vi "test-quintic-spline-00.vi"() -> (3 "Test Passed":bool)   [LabVIEW 2019]
uses:
  <vilib>/Rock Robotics/WPI/ThirdParty/JAS_Junk/TrajLib/POSEwCURVATURE.ctl
  <vilib>/Rock Robotics/WPI/ThirdParty/JAS_Junk/TrajLib/POSE2D.ctl
  <vilib>/Rock Robotics/WPI/ThirdParty/JAS_Junk/TrajLib/TRANSLATION2D.ctl
  <vilib>/Rock Robotics/WPI/ThirdParty/JAS_Junk/TrajLib/ROTATION2D.ctl
  <vilib>/Rock Robotics/WPI/ThirdParty/JAS_Junk/TrajLib/Rotation2d_CreateAngle.vi
  <vilib>/Rock Robotics/WPI/ThirdParty/JAS_Junk/TrajLib/Translation2d_Create.vi
  <vilib>/Rock Robotics/WPI/ThirdParty/JAS_Junk/TrajLib/Util_CalcDist.vi
  <vilib>/Rock Robotics/WPI/ThirdParty/JAS_Junk/TrajLib/Trajectory_Library.lvlib
panel:
  out "XY Graph":cluster{dbl[], dbl[]}(graph)
  out "Numb\nWaypoints":i32
  out "All Interior \nwayPoints\nFound (True)":bool
  out "end rot = 0":dbl
  out "end y = 0":dbl
  out "end x = 0":dbl
  out "start rot = 0":dbl
  out "start y = 0":dbl
  out "start x = 0":dbl
  out "max dtheta < 0.0872":dbl
  out "max dy < 0.00127":dbl
  out "max dx  < 0.127":dbl
  out "Overall Error":errorcluster
  out "Elements":i32
  out "Create Spline Error":errorcluster
  out "SplinePoses\nWCurve":T1[](array[typedef]) {"POSE"."ROTATION"."SIN" format="%13.4f"; "POSE"."ROTATION"."COS" format="%13.4f"; "POSE"."ROTATION"."VALUE" format="%13.4f"; "POSE"."TRANSLATION"."Y" format="%14.3f"; "POSE"."TRANSLATION"."X" format="%14.3f"}
  out "Elapsed Time":dbl
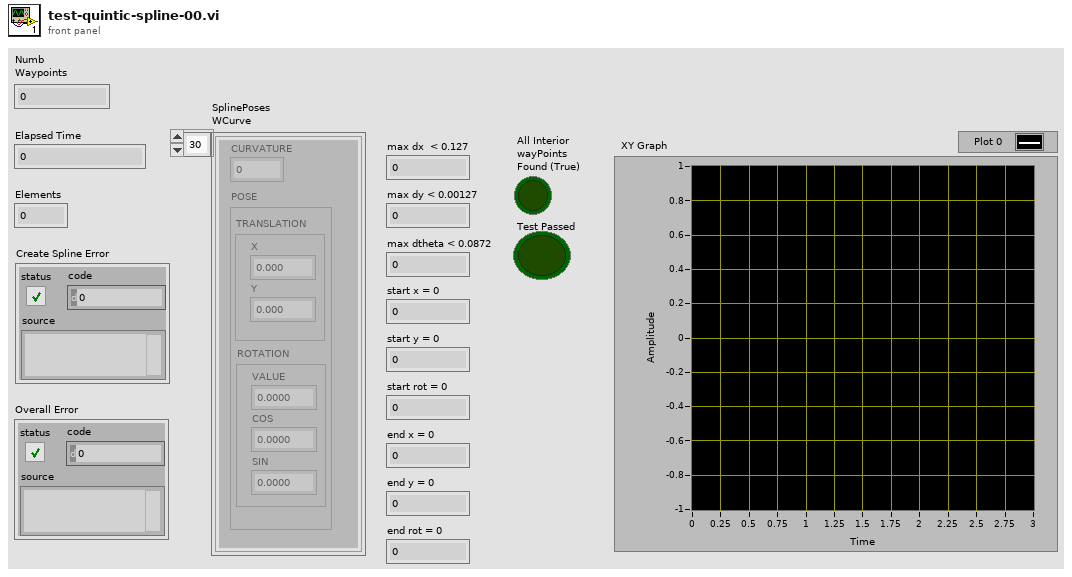
[diagram p1: front panel]
types:
  T1 = typedef "Trajectory_Library.lvlib/POSEwCURVATURE.ctl" = cluster{"CURVATURE":dbl, "POSE":T2}
  T2 = typedef "Trajectory_Library.lvlib/POSE2D.ctl" = cluster{"TRANSLATION":T3, "ROTATION":T4}
  T3 = typedef "Trajectory_Library.lvlib/TRANSLATION2D.ctl" = cluster{"X":dbl, "Y":dbl}
  T4 = typedef "Trajectory_Library.lvlib/ROTATION2D.ctl" = cluster{"VALUE":dbl, "COS":dbl, "SIN":dbl}
  T5 = typedef "Trajectory_Library.lvlib/SPLINE.ctl" = cluster{"Degree":i32, "Coefficients":T6}
  T6 = typedef "NI_Matrix.lvlib/RealMatrix.ctl" = dbl[][]
  T7 = typedef "Trajectory_Library.lvlib/TWIST2D.ctl" = cluster{"dX":dbl, "dY":dbl, "dTHETA":dbl}
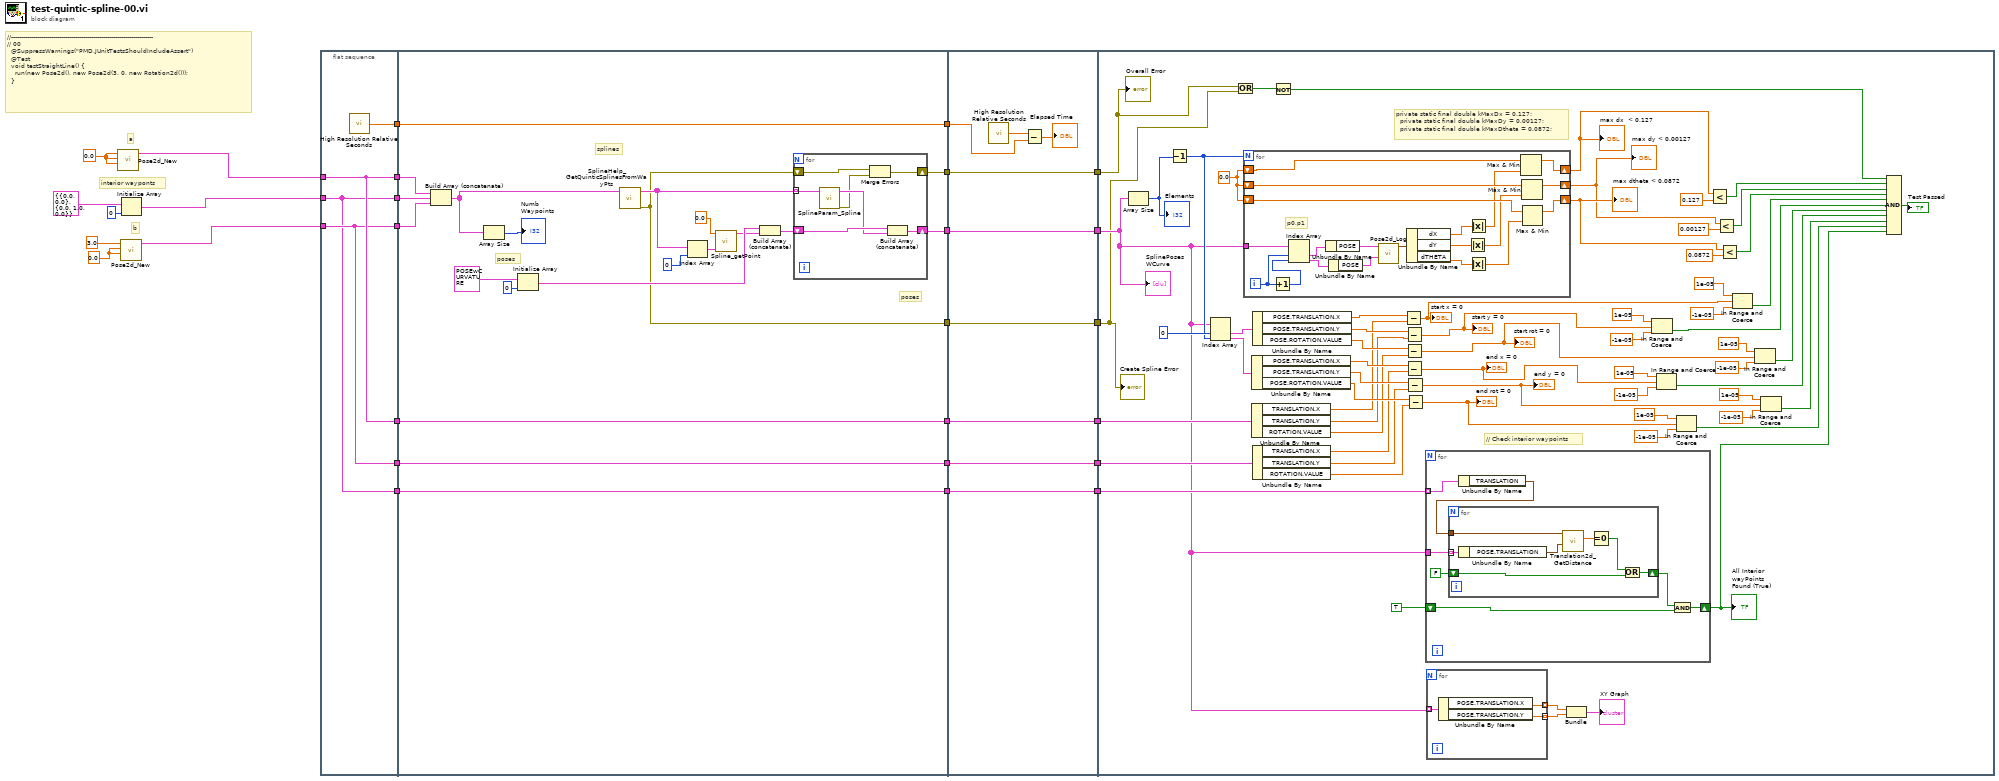
[diagram p0: block diagram]
diagram:
  w26 = 0.0 ("Y")
  w28 = 0.0 ("X")
  # "interior wayponts"
  # "b"
  # "a"
  # "//-----------------------------------------------------------------------\n// 00\n  @SuppressWarnings(\"PMD.JUnitTestsShouldIncludeAssert\")\n  @Test\n  void testStraightLine() {\n    run(new Pose2d(), new Pose2d(3, 0, new Rotation2d()));\n  }"
  n1 = call <vilib>:"Pose2d_New.vi"("Heading"=w28, "Y"=w28, "X"=w28) -> ("out POSe"=w25:T2)  [unwired: 8 in]
  n2 = call <vilib>:"Pose2d_New.vi"("Heading"=w26, "Y"=w26, "X"=3.0) -> ("out POSe"=w23:T2)  [unwired: 8 in]
  n3 = Initialize Array(T2 {"TRANSLATION"={"X"=0.0, "Y"=0.0}, "ROTATION"={"VALUE"=0.0, "COS"=1.0, "SIN"=0.0}} ("POSE"), 0 ("dimension size")) -> (w2:T2[])
  n4 = flat-sequence {
    tunnel: w25 -> [w31]
    tunnel: [w31] -> w24
    tunnel: w23 -> [w30]
    tunnel: [w30] -> w22
    tunnel: [w32] -> w21
    tunnel: [w31] -> w13
    tunnel: [w30] -> w10
    tunnel: [w29] -> w5
    tunnel: w2 -> [w29]
    tunnel: [w29] -> w1
    tunnel: w24 -> [w37]
    tunnel: w22 -> [w36]
    tunnel: [w53] -> w20
    tunnel: w21 -> [w53]
    tunnel: [w43] -> w19
    tunnel: [w42] -> w17
    tunnel: [w41] -> w15
    tunnel: w13 -> [w40]
    tunnel: [w40] -> w12
    tunnel: w10 -> [w39]
    tunnel: [w39] -> w9
    tunnel: [w38] -> w6
    tunnel: w5 -> [w38]
    tunnel: w1 -> [w35]
    tunnel: w20 -> [w69]
    tunnel: w19 -> [w68]
    tunnel: [w68] -> w18
    tunnel: w17 -> [w67]
    tunnel: [w67] -> w16
    tunnel: w15 -> [w66]
    tunnel: [w66] -> w14
    tunnel: w12 -> [w63]
    tunnel: [w63] -> w11
    tunnel: w9 -> [w62]
    tunnel: [w62] -> w8
    tunnel: [w61] -> w7
    tunnel: w6 -> [w61]
    tunnel: w18 -> [w110]
    tunnel: w16 -> [w97]
    tunnel: w14 -> [w96]
    tunnel: w11 -> [w132]
    tunnel: w8 -> [w131]
    tunnel: w7 -> [w114]
    frame #0 {
      n5 = call <vilib>:"High Resolution Relative Seconds.vi"() -> ("relative seconds"=w32:dbl)
    }
    frame #1 {
      # "poses"
      # "poses"
      # "splines"
      n6 = Build Array (concatenate)(w37, w35, w36) -> (w33:T2[])
      n7 = Array Size(array=w33) -> (size(s)=→"Numb\nWaypoints":i32)
      n8 = Initialize Array(T1 {"CURVATURE"=0.0, "POSE"={"TRANSLATION"={"X"=0.0, "Y"=0.0}, "ROTATION"={"VALUE"=0.0, "COS"=1.0, "SIN"=0.0}}} ("POSEwCURVATURE"), 0 ("dimension size")) -> (w47:T1[])
      n9 = call <vilib>:"SplineHelp_GetQuinticSplinesFromWayPts.vi"("WayPoints"=w33) -> ("out Error"=w42:errorcluster, "Splines"=w44:T5[])  [unwired: 9 in]
      n10 = Index Array(array=w44, index=0) -> (element=w49:T5)
      n11 = call <vilib>:"Spline_getPoint.vi"("inputSPLINE"=w49, "Time"=0.0) -> ("POSEwCURVATURE"=w46:T1)  [unwired: 9 in]
      n12 = Build Array (concatenate)(w47, w46) -> (w45:T1[])
      n13 = for {
        shift-right: [w57] -> w43
        shift-left: w45 -> [w59]
        tunnel: w44 -> [w60] mode=indexing
        shift-right: [w55] -> w41
        shift-left: w42 -> [w56]
        n14 = call <vilib>:"SplineParam_Spline.vi"("inputSPLINE"=w60) -> ("error out"=w54:errorcluster, "outputPOSEwCURVATURE"=w58:T1[])  [unwired: 9 in]
        n15 = Merge Errors(w56, w54) -> (w55:errorcluster)
        n16 = Build Array (concatenate)(w59, w58) -> (w57:T1[])
      }
    }
    frame #2 {
      n17 = call <vilib>:"High Resolution Relative Seconds.vi"() -> ("relative seconds"=w64:dbl)
      n18 = Subtract(x=w64, y=w69) -> (x-y=→"Elapsed Time":dbl)
    }
    frame #3 {
      w133 = 0.0
      # "// Check interior waypoints"
      # "private static final double kMaxDx = 0.127;\n  private static final double kMaxDy = 0.00127;\n  private static final double kMaxDtheta = 0.0872;"
      n19 = Array Size(array=w110) -> (size(s)=w134:i32)
      "Elements" <- w134
      n20 = Decrement(x=w134) -> (x-1=w129:i32)
      n21 = Index Array(array=w110, index #1=0 ("index"), index #2=w129) -> (element #1=w128:T1, element #2=w127:T1)
      n22 = Or(x=w96, y=w97) -> (x .or. y?=w98:bool)
      n23 = for {
        N: w129 -> [_]
        tunnel: w110 -> [w169]
        shift-right: [w160] -> w102
        shift-left: w133 -> [w157]
        shift-right: [w158] -> w104
        shift-left: w133 -> [w155]
        shift-right: [w159] -> w103
        shift-left: w133 -> [w156]
        i -> [w171]
        # "p0,p1"
        n24 = Increment(x=w171) -> (x+1=w170:i32)
        n25 = Index Array(array=w169, index #1=w171, index #2=w170) -> (element #1=w168:T1, element #2=w167:T1)
        n26 = Unbundle By Name(w168) -> ("POSE"=w166:T2)
        n27 = Unbundle By Name(w167) -> ("POSE"=w165:T2)
        n28 = call <vilib>:"Pose2d_Log.vi"("end POSE"=w165, "in POSE"=w166) -> ("out TWIST"=w164:T7)  [unwired: 9 in]
        n29 = Unbundle By Name(w164) -> ("dX"=w161:dbl, "dY"=w162:dbl, "dTHETA"=w163:dbl)
        n30 = Absolute Value(x=w162) -> (abs(x)=w153:dbl)
        n31 = Absolute Value(x=w161) -> (abs(x)=w154:dbl)
        n32 = Absolute Value(x=w163) -> (abs(x)=w152:dbl)
        n33 = Max & Min(x=w157, y=w154) -> (max(x,y)=w160:dbl)  [unwired: 1 out]
        n34 = Max & Min(x=w156, y=w153) -> (max(x,y)=w159:dbl)  [unwired: 1 out]
        n35 = Max & Min(x=w155, y=w152) -> (max(x,y)=w158:dbl)  [unwired: 1 out]
      }
      "max dx  < 0.127" <- w102
      "max dy < 0.00127" <- w103
      "max dtheta < 0.0872" <- w104
      n36 = Unbundle By Name(w127) -> ("POSE.TRANSLATION.X"=w123:dbl, "POSE.TRANSLATION.Y"=w122:dbl, "POSE.ROTATION.VALUE"=w121:dbl)
      n37 = Unbundle By Name(w132) -> ("TRANSLATION.X"=w120:dbl, "TRANSLATION.Y"=w119:dbl, "ROTATION.VALUE"=w118:dbl)
      n38 = Unbundle By Name(w128) -> ("POSE.TRANSLATION.X"=w126:dbl, "POSE.TRANSLATION.Y"=w125:dbl, "POSE.ROTATION.VALUE"=w124:dbl)
      n39 = Unbundle By Name(w131) -> ("TRANSLATION.X"=w117:dbl, "TRANSLATION.Y"=w116:dbl, "ROTATION.VALUE"=w115:dbl)
      n40 = Not(x=w98) -> (.not. x?=w95:bool)
      n41 = Subtract(x=w126, y=w120) -> (x-y=w91:dbl)
      "start x = 0" <- w91
      n42 = Subtract(x=w125, y=w119) -> (x-y=w70:dbl)
      "start y = 0" <- w70
      n43 = Subtract(x=w124, y=w118) -> (x-y=w74:dbl)
      "start rot = 0" <- w74
      n44 = Subtract(x=w123, y=w117) -> (x-y=w75:dbl)
      "end x = 0" <- w75
      n45 = Subtract(x=w122, y=w116) -> (x-y=w82:dbl)
      "end y = 0" <- w82
      n46 = Subtract(x=w121, y=w115) -> (x-y=w86:dbl)
      "end rot = 0" <- w86
      n47 = for {
        tunnel: w114 -> [w139] mode=indexing
        tunnel: w110 -> [w144]
        shift-right: [w143] -> w94
        shift-left: TRUE -> [w142]
        n48 = Unbundle By Name(w139) -> ("TRANSLATION"=w138:T3)
        n49 = for {
          tunnel: w144 -> [w148] mode=indexing
          shift-right: [w151] -> w140
          shift-left: FALSE -> [w150]
          tunnel: w138 -> [w149]
          n50 = Unbundle By Name(w148) -> ("POSE.TRANSLATION"=w147:T3)
          n51 = call <vilib>:"Translation2d_GetDistance.vi"("other Translation"=w147, "In Translation"=w149) -> ("Distance"=w146:dbl)  [unwired: 9 in]
          n52 = Equal To 0?(x=w146) -> (x = 0?=w145:bool)
          n53 = Or(x=w145, y=w150) -> (x .or. y?=w151:bool)
        }
        n54 = And(x=w140, y=w142) -> (x .and. y?=w143:bool)
      }
      "All Interior \nwayPoints\nFound (True)" <- w94
      n55 = for {
        tunnel: [w137] -> w112 mode=indexing
        tunnel: [w136] -> w111 mode=indexing
        tunnel: w110 -> [w135] mode=indexing
        n56 = Unbundle By Name(w135) -> ("POSE.TRANSLATION.X"=w137:dbl, "POSE.TRANSLATION.Y"=w136:dbl)
      }
      n57 = Bundle(w112, w111) -> (→"XY Graph":cluster{dbl[], dbl[]})  [unwired: 1 in]
      n58 = In Range and Coerce(upper limit=1e-05, x=w70, lower limit=-1e-05) -> (In Range?=w71:bool)  [unwired: 1 out]
      n59 = In Range and Coerce(upper limit=1e-05, x=w75, lower limit=-1e-05) -> (In Range?=w77:bool)  [unwired: 1 out]
      n60 = In Range and Coerce(upper limit=1e-05, x=w86, lower limit=-1e-05) -> (In Range?=w87:bool)  [unwired: 1 out]
      n61 = Less?(x=w102, y=0.127) -> (x < y?=w101:bool)
      n62 = Less?(x=w103, y=0.00127) -> (x < y?=w100:bool)
      n63 = Less?(x=w104, y=0.0872) -> (x < y?=w99:bool)
      n64 = In Range and Coerce(upper limit=1e-05, x=w91, lower limit=-1e-05) -> (In Range?=w90:bool)  [unwired: 1 out]
      n65 = In Range and Coerce(upper limit=1e-05, x=w74, lower limit=-1e-05) -> (In Range?=w76:bool)  [unwired: 1 out]
      n66 = In Range and Coerce(upper limit=1e-05, x=w82, lower limit=-1e-05) -> (In Range?=w83:bool)  [unwired: 1 out]
      n67 = Compound Arithmetic op=AND(w95, w101, w100, w99, w90, w71, w76, w77, w83, w87, w94) -> (→"Test Passed":bool)
      "SplinePoses\nWCurve" <- w110
      "Create Spline Error" <- w97
      "Overall Error" <- w96
    }
  }
